vi "Close.vi"(8 "error in":errorcluster, 11 "Custom Events in":refnum<class "Custom Events.lvclass">) -> (0 "error out":errorcluster, 3 "Custom Events out":refnum<class "Custom Events.lvclass">)   [LabVIEW 2024, in "SourceGrid.lvlib" / "Custom Events.lvclass"]
uses:
  Custom Events.lvclass
  Custom Events.lvclass/Custom Events.ctl
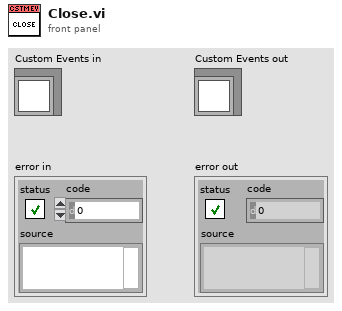
[diagram p1: front panel]
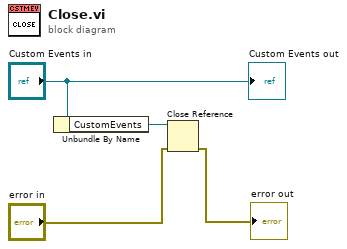
[diagram p0: block diagram]
diagram:
  n1 = Unbundle By Name("Custom Events in") -> ("CustomEvents"=w3:refnum<k24>)
  n2 = Close Reference(reference=w3, error in (no error)="error in") -> (error out=→"error out":errorcluster)
  "Custom Events out" <- "Custom Events in"
